vi "Write Environment Options.vi"(8 "error in (no error)":errorcluster, 10 "Environment Options":T1, 11 "WebView2 Control in":refnum<class "WebView2 QControl.lvclass">) -> (0 "error out":errorcluster, 3 "WebView2 Control out":refnum<class "WebView2 QControl.lvclass">)   [LabVIEW 2020, in "WebView2 QControl.lvlib" / "WebView2 QControl.lvclass"]
uses:
  WebView2 QControl.lvclass
  Webview2 Lib/WebView2 Control Object/Core Env Options.ctl
  WebView2 QControl.lvclass/WebView2 QControl.ctl
  Webview2 Lib/WebView2 Control Object/WebView2 Control.lvclass
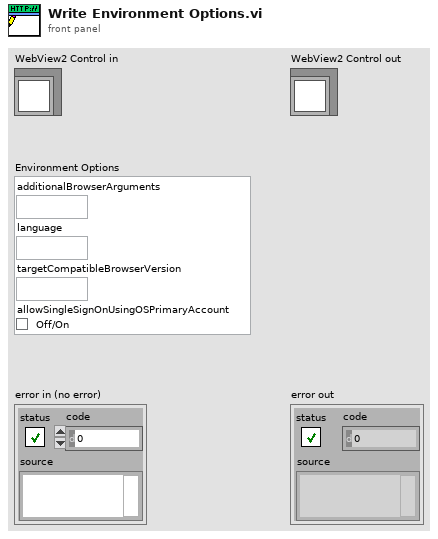
[diagram p1: front panel]
types:
  T1 = typedef "WebView2.lvlib/WebView2 Control.lvclass/Core Env Options.ctl" = cluster{"additionalBrowserArguments":string, "language":string, "targetCompatibleBrowserVersion":string, "allowSingleSignOnUsingOSPrimaryAccount":bool}
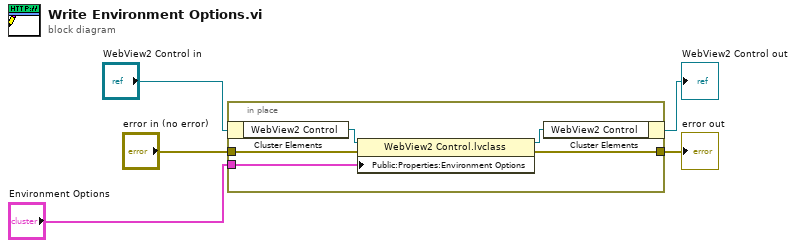
[diagram p0: block diagram]
diagram:
  n1 = in-place {
    in-place-border: "error in (no error)" -> [w10]
    in-place-border: [w9] -> w3
    in-place-border: "Environment Options" -> [w6]
    n2 = in-place-cluster #1("WebView2 Control in") -> ("WebView2 Control"=w8:refnum<class "WebView2 Control.lvclass">)
    n3 = property class="WebView2 Control.lvclass"(reference=w8, error in=w10, "Public:Properties:Environment Options"=w6) -> (reference out=w7:refnum<class "WebView2 Control.lvclass">, error out=w9:errorcluster)
    n4 = in-place-cluster #1("WebView2 Control"=w7) -> (→"WebView2 Control out":refnum<class "WebView2 QControl.lvclass">)
  }
  "error out" <- w3
